vi "João aula 5.vi"() -> ()   [LabVIEW 2024]
uses:
  <vilib>/LabVIEW Open Source Project/Epoch Date & Time/epoch.UNIX/Epoch.UNIX.lvclass
panel:
  in  "stop":bool
  out "output waveform":waveform(dbl)
  out "Waveform Chart 2":waveform(dbl)(graph)
  out "Waveform Chart":dbl(graph)
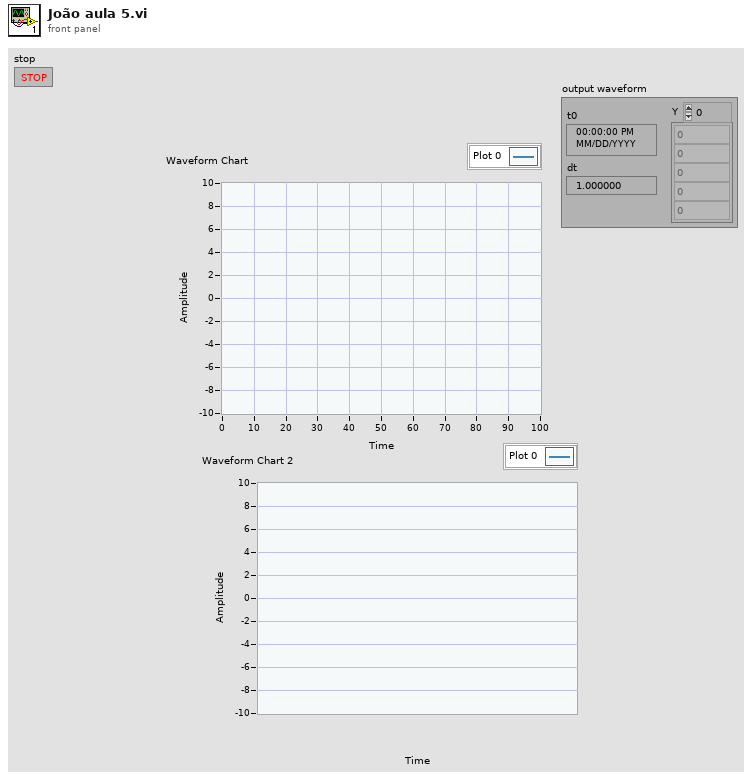
[diagram p1: front panel]
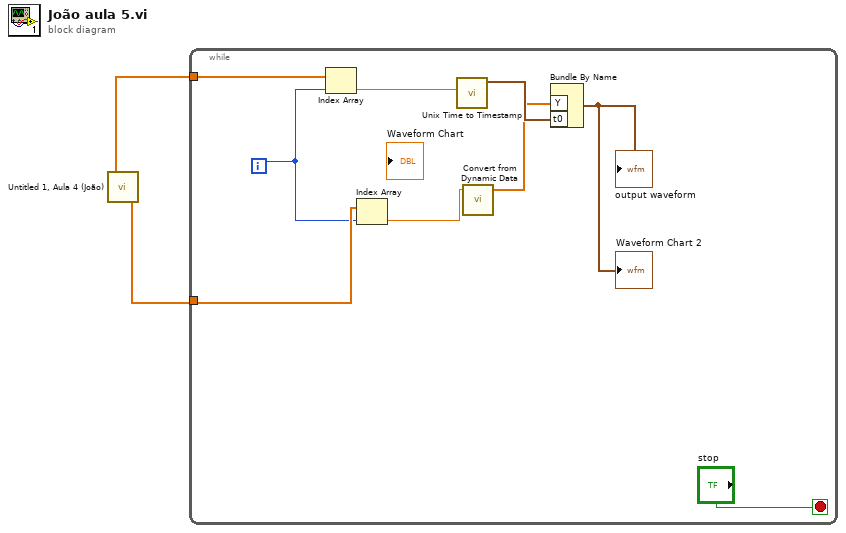
[diagram p0: block diagram]
diagram:
  n1 = call "Untitled 1, Aula 4 (João).vi"() -> ("Potencia ativa A"=w2:dbl[], "timestamp"=w1:dbl[])  [unwired: 2 out]
  n2 = while {
    tunnel: w2 -> [w11]
    tunnel: w1 -> [w10]
    i -> [w9]
    stop <- "stop" stop-if-true
    n3 = Index Array(array=w10, index=w9) -> (element=w8:dbl)
    n4 = Index Array(array=w11, index=w9) -> (element=w5:dbl)
    n5 = call <vilib>:"Unix Time to Timestamp.vi"("Fractional Second"=w8) -> ("Timestamp"=w7:timestamp)  [unwired: 9 in, 1 out]
    n6 = call "Convert from Dynamic Data"("Dynamic Data Type"=w5) -> ("Array"=w6:dbl[])  [unwired: 3 in]
    n7 = Bundle By Name("Y"=w6, "t0"=w7) -> (→"Waveform Chart 2" →"output waveform":waveform(dbl))  [unwired: 1 in]
  }
